vi "Control Panel No Objects.vi"() -> (0 "error out":errorcluster)   [LabVIEW 2009]
doc: "(Dynamic) A user-level application that simulates the physical front panel of the Instrument. Provide the user with buttons to manually control features of the instrument, and provide indicators of its current state."
uses:
  Global/GPIB Numbers.vi
  Fluke 8840/Fluke 8840.lvlib
panel:
  out "AutoRange":bool
  out "unit":string
  in  "Reset":bool
  in  "Read Current Value":bool
  out "Value":dbl
  in  "Set":bool
  in  "Read to Control":bool
  in  "Read":bool
  in  "trigger mode set":u16(ring) items=["internal - continuous trigger", "external - rear panel trigger with delay", "external - bus trigger with delay", "external - rear panel trigger", "external - bus trigger"]
  in  "rate set":u16(ring) items=["slow", "medium", "fast"]
  in  "range set":u16(ring)=6 items=["autorange", "200mV, 200 ohms", "2V, 2 kohms", "20V, 20 kohms", "200V, 200 kohms", "1000Vdc, 700 Vac, 2 Mohms", "20 Mohms"]
  in  "function set":u16(ring) items=["volts DC", "volts AC", "2-wire k.ohms", "4-wire k.ohms", "mA DC", "mA AC"]
  out "trigger mode":u16(ring) items=["internal - continuous trigger", "external - rear panel trigger with delay", "external - bus trigger with delay", "external - rear panel trigger", "external - bus trigger"]
  out "rate":u16(ring) items=["slow", "medium", "fast"]
  out "range":u16(ring)=6 items=["autorange", "200mV, 200 ohms", "2V, 2 kohms", "20V, 20 kohms", "200V, 200 kohms", "1000Vdc, 700 Vac, 2 Mohms", "20 Mohms"]
  out "function":u16(ring) items=["volts DC", "volts AC", "2-wire k.ohms", "4-wire k.ohms", "mA DC", "mA AC"]
  in  "stop":bool
  in  "Copy actual to set":bool
  in  "Populate fields with member data":bool
  # "Note: can't set trigger mode yet. Apparently need to create driver for the Y1 command"
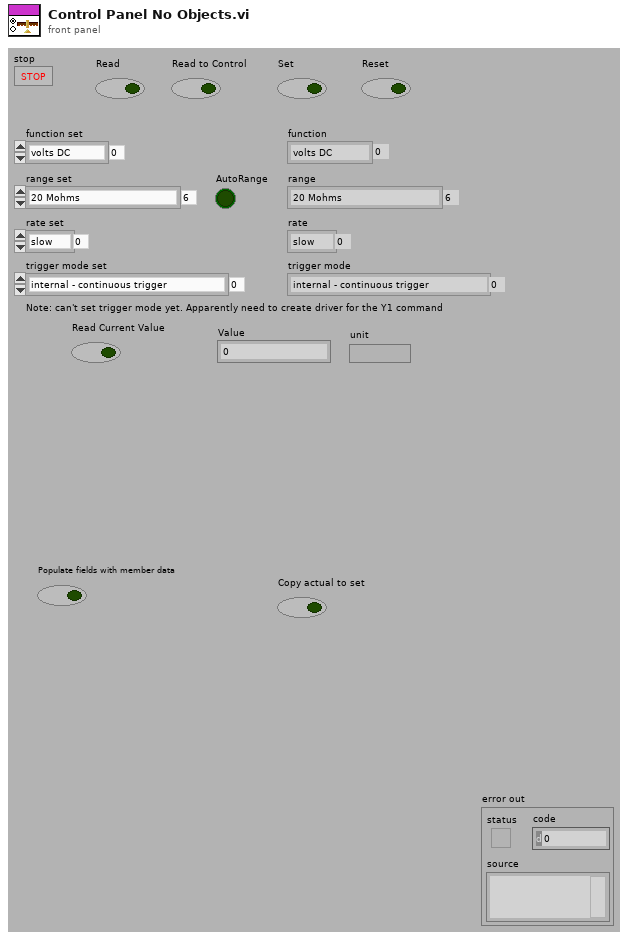
[diagram p1: front panel]
types:
  T1 = cluster{"function (0:volts DC)":i16, "range (0:auto)":i16, "rate (0:slow)":i16, "trigger mode (0:internal)":i16, "Autorange":bool}
  T2 = typedef "GPIB Type Def.ctl" = cluster{"Name":string, "bus":dbl, "GPIB":dbl, "GPIB as string":string, "byte":i32, "VISA Resource Name":refnum<visa-resource-name>}
  T3 = cluster{"function (0:volts DC)":i16, "range (0:auto)":i16, "rate (0:slow)":i16, "trigger mode (0:internal":i16, "Autorange":bool}
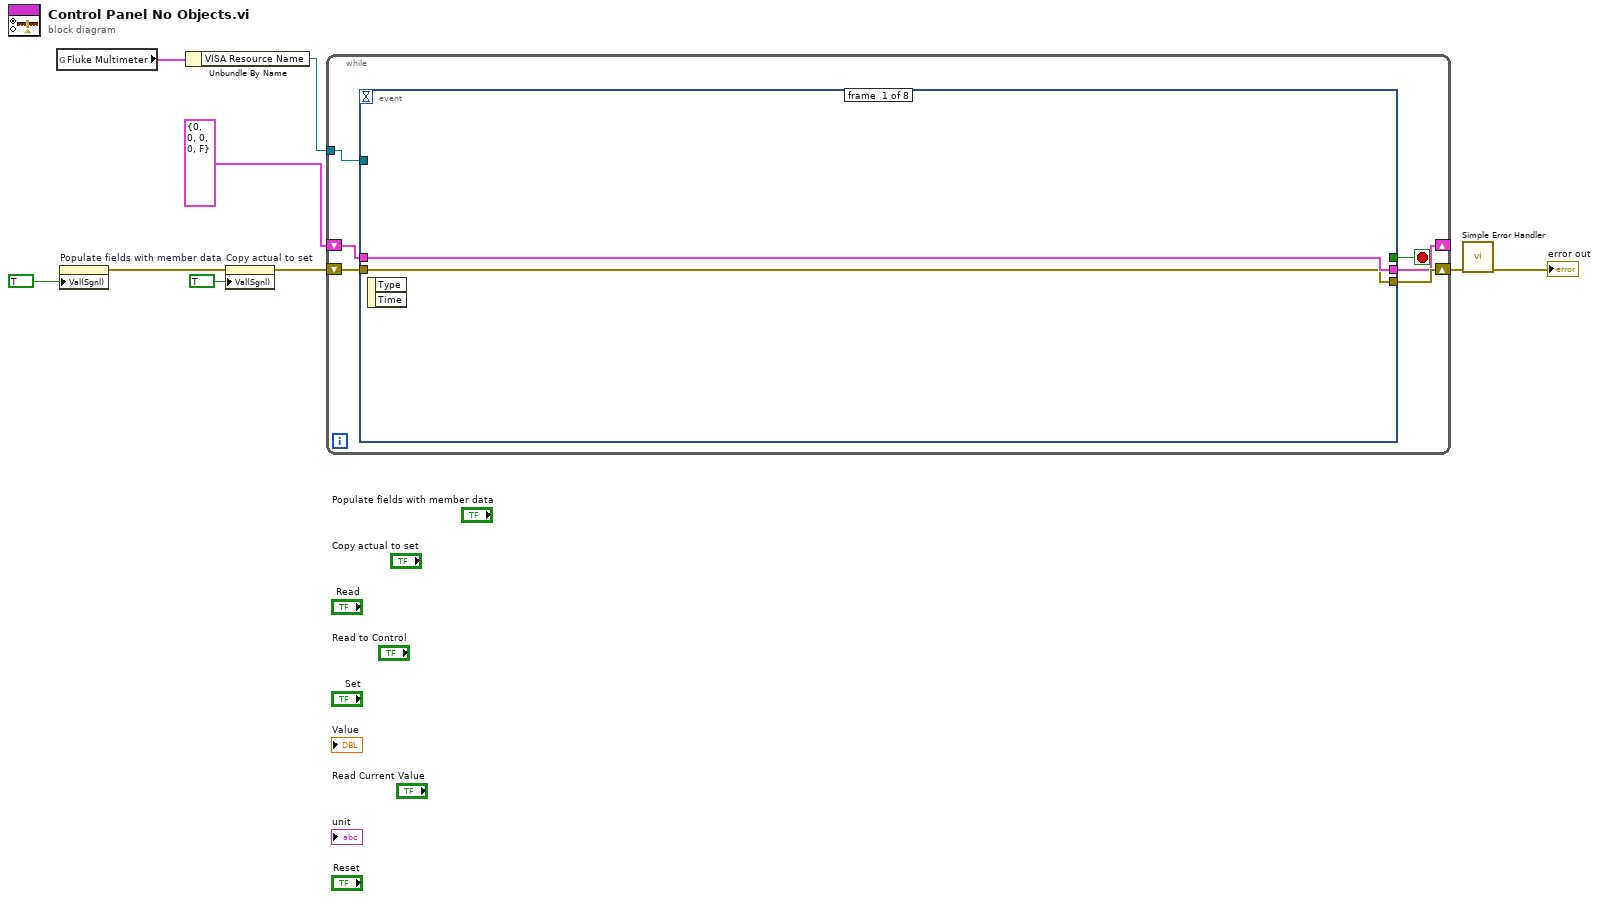
[diagram p0: block diagram]
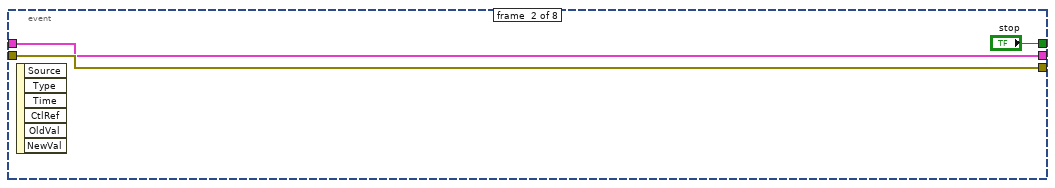
[diagram p2: hidden frame]
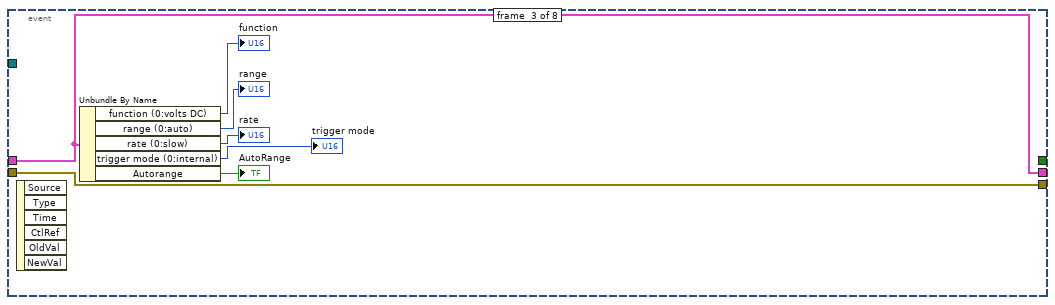
[diagram p3: hidden frame]
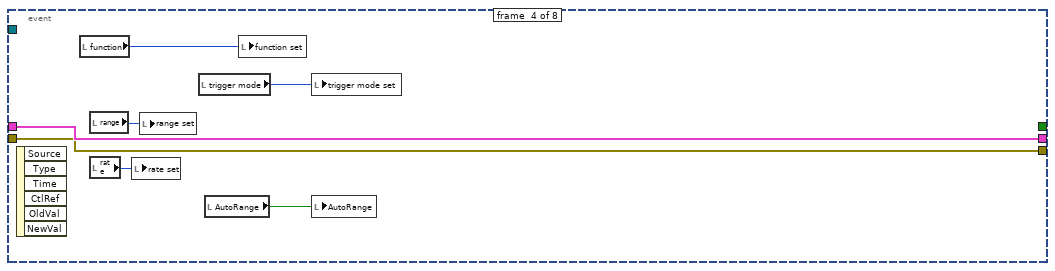
[diagram p4: hidden frame]
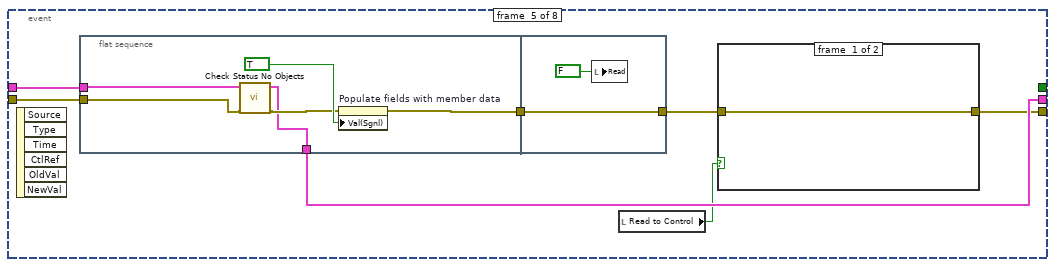
[diagram p5: hidden frame]
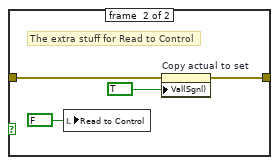
[diagram p6: hidden frame]
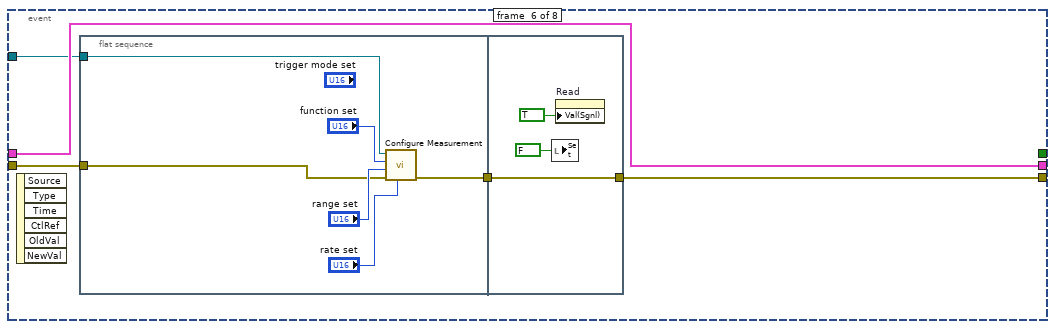
[diagram p7: hidden frame]
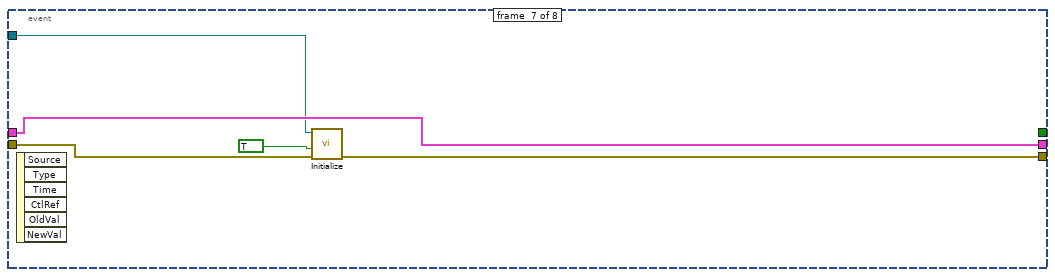
[diagram p8: hidden frame]
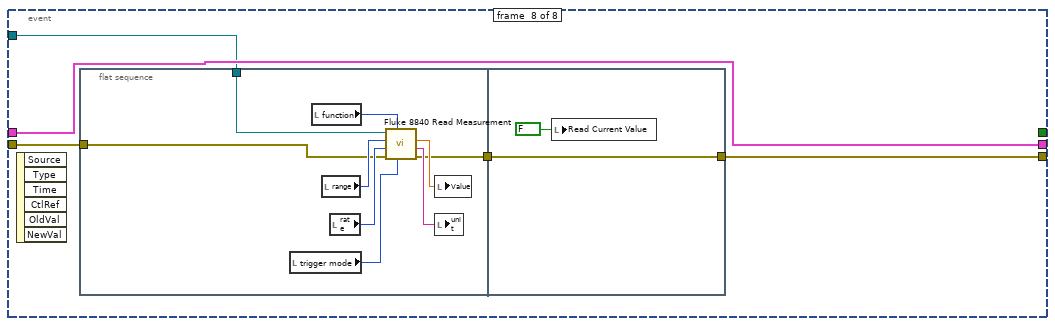
[diagram p9: hidden frame]
diagram:
  n1 = global read "GPIB Numbers.vi" "Fluke Multimeter"() -> (w2:T2)
  n2 = property on="Populate fields with member data" class="Bool (strict)"("Val(Sgnl)"=TRUE ("Value (Signaling)")) -> (error out=w9:errorcluster)  [unwired: 2 in, 1 out]
  n3 = Unbundle By Name(w2) -> ("VISA Resource Name"=w1:refnum<visa-resource-name>)
  n4 = property on="Copy actual to set" class="Bool (strict)"(error in=w9, "Val(Sgnl)"=TRUE ("Value (Signaling)")) -> (error out=w8:errorcluster)  [unwired: 1 in, 1 out]
  n5 = while {
    shift-right: [w12] -> _
    shift-left: T1 {"function (0:volts DC)"=0, "range (0:auto)"=0, "rate (0:slow)"=0, "trigger mode (0:internal)"=0, "Autorange"=FALSE} ("Initialize Cluster") -> [w11]
    shift-right: [w14] -> w5
    shift-left: w8 -> [w13]
    tunnel: w1 -> [w10]
    stop <- w15 stop-if-true
    n6 = event shown="[4] \"Read\", \"Read to Control\": Value Change" {
      selector: _ -> [_ _ _ _ _ _ _ _]
      dyn-events: _ -> [_ _ _ _ _ _ _ _]
      timeout: _ -> [_ _ _ _ _ _ _ _]
      tunnel: [_ "stop" _ _ _ _ _ _] -> w15
      tunnel: [w16 w19 w22 w29 w35 w58 w70 w78] -> w14
      tunnel: w13 -> [w16 w19 w22 w29 w41 w59 w71 w77]
      tunnel: [w17 w18 w23 w30 w39 w56 w72 w76] -> w12
      tunnel: w11 -> [w17 w18 w23 w30 w40 w56 w72 w76]
      tunnel: w10 -> [_ _ _ _ _ w55 w69 w74]
      event #0 {
        n7 = event-data() -> ()  [unwired: 3 out]
      }
      event #1 {
        n8 = event-data() -> ()  [unwired: 7 out]
      }
      event #2 {
        n9 = event-data() -> ()  [unwired: 7 out]
        n10 = Unbundle By Name(w23) -> ("function (0:volts DC)"=→"function":i16, "range (0:auto)"=→"range":i16, "rate (0:slow)"=→"rate":i16, "trigger mode (0:internal)"=→"trigger mode":i16, "Autorange"=→"AutoRange":bool)
      }
      event #3 {
        n11 = event-data() -> ()  [unwired: 7 out]
        n12 = local read "function"() -> (w34:u16)
        n13 = local read "range"() -> (w33:u16)
        n14 = local read "rate"() -> (w32:u16)
        n15 = local write "rate set"(w32) -> ()
        n16 = local write "range set"(w33) -> ()
        n17 = local read "trigger mode"() -> (w31:u16)
        n18 = local read "AutoRange"() -> (w28:bool)
        n19 = local write "function set"(w34) -> ()
        n20 = local write "trigger mode set"(w31) -> ()
        n21 = local write "AutoRange"(w28) -> ()
      }
      event #4 {
        n22 = event-data() -> ()  [unwired: 7 out]
        n23 = flat-sequence {
          tunnel: w41 -> [w49]
          tunnel: w40 -> [w48]
          tunnel: [w47] -> w39
          tunnel: [w51] -> w36
          tunnel: [w53] -> w37
          tunnel: w36 -> [w53]
          frame #0 {
            n24 = call "Check Status No Objects.vi"("error in (no error)"=w49, "input cluster"=w48) -> ("error out"=w50:errorcluster, "output cluster"=w47:T3)  [unwired: 6 in, 2 out]
            n25 = property on="Populate fields with member data" class="Bool (strict)"(error in=w50, "Val(Sgnl)"=TRUE ("Value (Signaling)")) -> (error out=w51:errorcluster)  [unwired: 1 in, 1 out]
          }
          frame #1 {
            n26 = local write "Read"(FALSE ("Read")) -> ()
          }
        }
        n27 = local read "Read to Control"() -> (w38:bool)
        n28 = case shown="True" w38 {
          tunnel: w37 -> [w42 w44]
          tunnel: [w42 w43] -> w35
          frame #0 {
          }
          frame #1 {
            # "The extra stuff for Read to Control"
            n29 = local write "Read to Control"(FALSE ("Read to Control")) -> ()
            n30 = property on="Copy actual to set" class="Bool (strict)"(error in=w44, "Val(Sgnl)"=TRUE ("Value (Signaling)")) -> (error out=w43:errorcluster)  [unwired: 1 in, 1 out]
          }
        }
      }
      event #5 {
        n31 = event-data() -> ()  [unwired: 7 out]
        n32 = flat-sequence {
          tunnel: w59 -> [w61]
          tunnel: [w62] -> w57
          tunnel: w55 -> [w60]
          tunnel: [w68] -> w58
          tunnel: w57 -> [w68]
          frame #0 {
            n33 = call "Configure Measurement.vi"("rate (0:slow)"="rate set", "error in (no error)"=w61, "range (0:auto)"="range set", "function (0:volts DC)"="function set", "VISA resource name"=w60) -> ("error out"=w62:errorcluster)  [unwired: 6 out]
          }
          frame #1 {
            n34 = local write "Set"(FALSE ("Set")) -> ()
            n35 = property on="Read" class="Bool (strict)"("Val(Sgnl)"=TRUE ("Value (Signaling)")) -> ()  [unwired: 2 in, 2 out]
          }
        }
      }
      event #6 {
        n36 = event-data() -> ()  [unwired: 7 out]
        n37 = call "Initialize.vi"("error in (no error)"=w71, "reset (T:yes)"=TRUE, "VISA resource name"=w69) -> ("error out"=w70:errorcluster)  [unwired: 8 out]
      }
      event #7 {
        n38 = event-data() -> ()  [unwired: 7 out]
        n39 = flat-sequence {
          tunnel: w77 -> [w80]
          tunnel: [w81] -> w75
          tunnel: w74 -> [w79]
          tunnel: [w89] -> w78
          tunnel: w75 -> [w89]
          frame #0 {
            n40 = local read "trigger mode"() -> (w87:u16)
            n41 = local read "function"() -> (w84:u16)
            n42 = local read "range"() -> (w85:u16)
            n43 = local read "rate"() -> (w86:u16)
            n44 = call "Fluke 8840 Read Measurement.vi"("trigger mode (0:internal)"=w87, "function (0:volts DC)"=w84, "error in (no error)"=w80, "rate (0:slow)"=w86, "range (0:auto)"=w85, "VISA resource name"=w79) -> ("error out"=w81:errorcluster, "unit"=w82:string, "measurement"=w83:dbl)  [unwired: 3 out]
            n45 = local write "Value"(w83) -> ()
            n46 = local write "unit"(w82) -> ()
          }
          frame #1 {
            n47 = local write "Read Current Value"(FALSE ("Read Current Value")) -> ()
          }
        }
      }
    }
  }
  n48 = call <vilib>:"Simple Error Handler.vi"("error in (no error)"=w5) -> ("error out"=→"error out":errorcluster)  [unwired: 1 in, 7 out]
